vi "CreateReferences.vi"(8 "error in (no error)":errorcluster, 11 "Connection in":refnum<class "Connection.lvclass">) -> (0 "error out":errorcluster, 3 "Connection out":refnum<class "Connection.lvclass">)   [LabVIEW 2013, in "MQTT_Connection.lvlib" / "Connection.lvclass"]
uses:
  Connection.lvclass
  Connection.lvclass/Connection.ctl
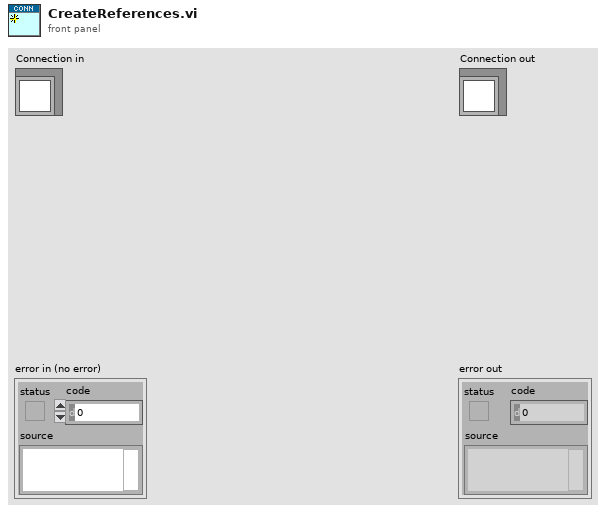
[diagram p1: front panel]
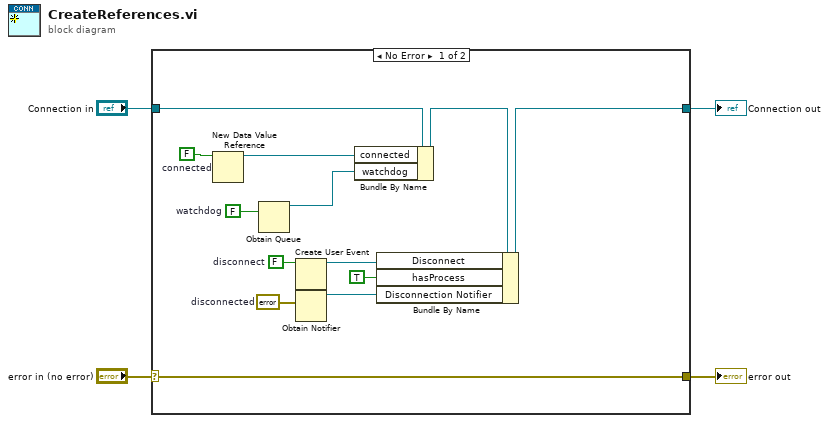
[diagram p0: block diagram]
diagram:
  n1 = case shown="No Error" "error in (no error)" {
    selector: "error in (no error)" -> [w16 w19]
    tunnel: [w16 w19] -> w3
    tunnel: [w5 w18] -> w1
    tunnel: "Connection in" -> [w17 w18]
    frame No Error {
      w7 = errorcluster {"status"=FALSE, "code"=0, "source"=""}  # disconnected
      w11 = FALSE  # disconnect
      w13 = FALSE  # watchdog
      w15 = FALSE  # connected
      n2 = New Data Value Reference(data value=w15) -> (data value reference=w14:refnum<data-value>)  [unwired: 1 in, 1 out]
      n3 = Obtain Queue(element data type=w13) -> (queue out=w12:refnum<queue>)  [unwired: 4 in, 2 out]
      n4 = Create User Event(user event datatype=w11) -> (user event=w10:refnum<user-event>)  [unwired: 1 in, 1 out]
      n5 = Obtain Notifier(notification data type=w7) -> (notifier out=w8:refnum<notifier>)  [unwired: 3 in, 2 out]
      n6 = Bundle By Name(cluster=w17, "connected"=w14, "watchdog"=w12) -> (w6:refnum<class "Connection.lvclass">)
      n7 = Bundle By Name(cluster=w6, "Disconnect"=w10, "hasProcess"=TRUE, "Disconnection Notifier"=w8) -> (w5:refnum<class "Connection.lvclass">)
    }
    frame Error {
    }
  }
  "error out" <- w3
  "Connection out" <- w1
